vi "FP Server Set Data.vi"(8 "error in (no error)":errorcluster, 10 "Data":string[][](array[string]), 11 "Page":string) -> (0 "error out":errorcluster)   [LabVIEW 2017, in "Front Panel Publisher.lvlib" / "Front Panel Manager.lvclass"]
uses:
  Front Panel Manager.lvclass
  Protected/FP Server Message.ctl
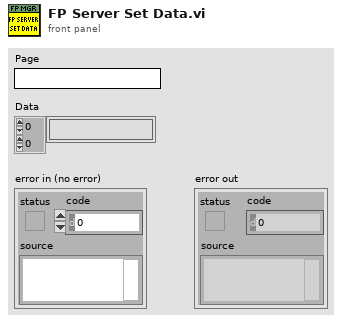
[diagram p1: front panel]
types:
  T1 = typedef "Front Panel Publisher.lvlib/Front Panel Manager.lvclass/FP Server Message.ctl" = cluster{"Message":string, "Page":string, "Data":string[][], "Connection ID":u64, "Values and Position":refnum<vi>[]}
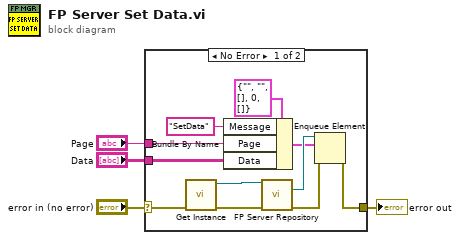
[diagram p0: block diagram]
diagram:
  n1 = case shown="No Error" "error in (no error)" {
    selector: "error in (no error)" -> [w12 w16]
    tunnel: [w5 w16] -> w3
    tunnel: "Page" -> [w7 _]
    tunnel: "Data" -> [w6 _]
    frame No Error {
      n2 = call "Get Instance.vi"("error in (no error)"=w12) -> ("error out"=w11:errorcluster, "FP Manager Out"=w13:refnum<class "Front Panel Manager.lvclass">)  [unwired: 6 in, 3 out]
      n3 = Bundle By Name(cluster=T1 {"Message"="", "Page"="", "Data"=[], "Connection ID"=0, "Values and Position"=[]} ("element"), "Message"="SetData", "Page"=w7, "Data"=w6) -> (w9:T1)
      n4 = call "FP Server Repository.vi"("FP Management In"=w13, "error in (no error)"=w11) -> ("ToProcessQueue"=w10:refnum<queue>, "error out"=w14:errorcluster)  [unwired: 7 in, 5 out]
      n5 = Enqueue Element(queue=w10, element=w9, error in (no error)=w14) -> (error out=w5:errorcluster)  [unwired: 1 in, 2 out]
    }
    frame Error {
    }
  }
  "error out" <- w3
